vi "GTH-V2.MISC.vi"(7 "CMD":enum16{"All", "ChanA", "ChanB", "Single"}(ring), 8 "Error In":errorcluster caption="错误输入", 9 "ON/FF":bool, 10 "Para":T1(ring), 11 "VISA资源输入":refnum<visa-resource-name>) -> (0 "Error Out":errorcluster caption="错误输出", 2 "CMD Info":string, 3 "OK?":bool)   [LabVIEW 2012, in "Lib_UEL.ATE.lvlib" / "STM32-CoreBD.lvlib"]
uses:
  STM32-CoreBD.lvlib
panel:
  out "Return":string
  # "Version History\nV1.0.0,2015-8-11, 适用于新版GTH-V2硬件."
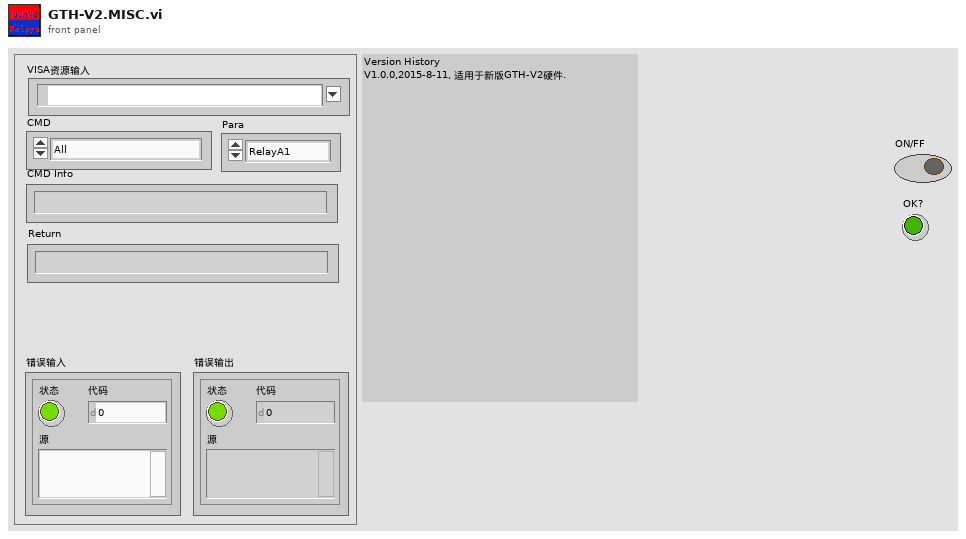
[diagram p1: front panel]
types:
  T1 = enum16{"RelayA1", "RelayA2", "RelayA3", "RelayA4", "RelayA5", "RelayA6", "RelayA7", "RelayA8", "RelayA9", "RelayA10", "RelayB1", "RelayB2", "RelayB3", "RelayB4", "RelayB5", "RelayB6", "RelayB7", "RelayB8", "RelayB9", "RelayB10", "ADC1", "ADC2", "ADC3", "DAC1"}
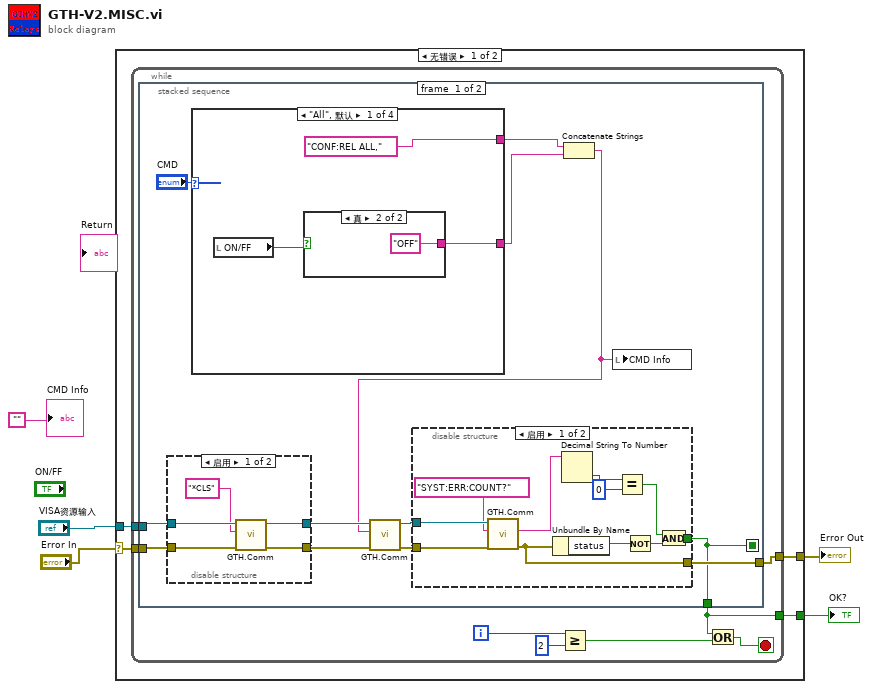
[diagram p0: block diagram]
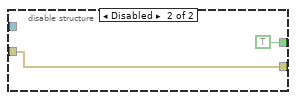
[diagram p2: hidden frame]
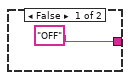
[diagram p4: hidden frame]
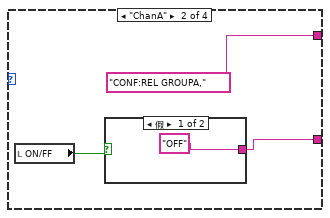
[diagram p5: hidden frame]
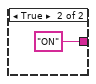
[diagram p6: hidden frame]
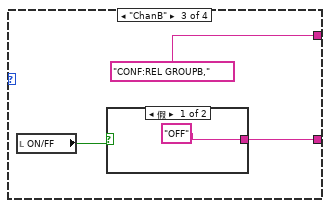
[diagram p7: hidden frame]
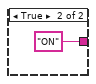
[diagram p8: hidden frame]
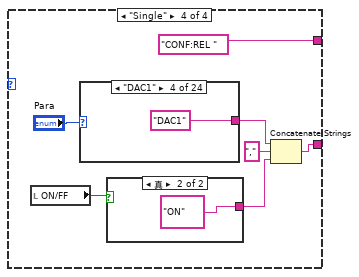
[diagram p9: hidden frame]
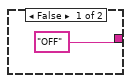
[diagram p10: hidden frame]
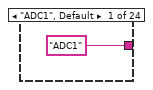
[diagram p11: hidden frame]
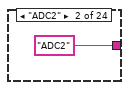
[diagram p12: hidden frame]
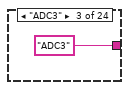
[diagram p13: hidden frame]
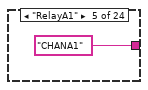
[diagram p14: hidden frame]
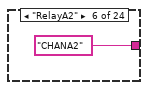
[diagram p15: hidden frame]
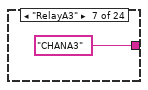
[diagram p16: hidden frame]
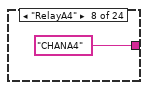
[diagram p17: hidden frame]
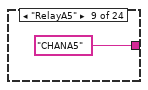
[diagram p18: hidden frame]
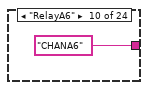
[diagram p19: hidden frame]
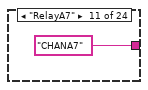
[diagram p20: hidden frame]
diagram:
  n1 = case shown="无错误" "Error In" {
    selector: "Error In" -> [w8 w101]
    tunnel: [w7 w101] -> w5
    tunnel: "VISA资源输入" -> [w9 _]
    tunnel: [w6 FALSE] -> w1
    frame No Error {
      n2 = while {
        tunnel: w9 -> [w17]
        tunnel: w8 -> [w16]
        tunnel: [w15] -> w7
        tunnel: [w10] -> w6
        i -> [w13]
        stop <- w14 stop-if-true
        n3 = stacked-sequence {
          seq-local: [w18 _] -> [_ w98]
          tunnel: w17 -> [w27 _]
          tunnel: w16 -> [w26 _]
          tunnel: [w19 _] -> w15
          tunnel: [w18 _] -> w10
          frame #0 {
            n4 = disable-structure shown="启用" {
              disable-tunnel: w27 -> [w47 w49]
              disable-tunnel: w26 -> [w46 w48]
              disable-tunnel: [w44 w49] -> w25
              disable-tunnel: [w43 w48] -> w24
              frame Enabled {
                n5 = call "GTH.Comm.vi"("Error In"=w46, "SCPI CMD"="*CLS", "USB Port In"=w47) -> ("Error Out"=w43:errorcluster, "USB Port Out"=w44:refnum<visa-resource-name>)  [unwired: 3 in, 4 out]
              }
              frame Disabled {
              }
            }
            n6 = case shown="\"All\", 默认" "CMD" {
              tunnel: ["CONF:REL ALL," ("字符串") "CONF:REL GROUPA," ("字符串") "CONF:REL GROUPB," ("字符串") "CONF:REL " ("字符串")] -> w23
              tunnel: [w51 w55 w60 w68] -> w28
              frame "All", Default {
                n7 = local read "ON/FF"() -> (w50:bool)
                n8 = case shown="真" w50 {
                  tunnel: ["OFF" ("字符串") "OFF" ("字符串")] -> w51
                  frame False {
                  }
                  frame True {
                  }
                }
              }
              frame "ChanA" {
                n9 = local read "ON/FF"() -> (w56:bool)
                n10 = case shown="假" w56 {
                  tunnel: ["OFF" ("字符串") "ON" ("字符串")] -> w55
                  frame False {
                  }
                  frame True {
                  }
                }
              }
              frame "ChanB" {
                n11 = local read "ON/FF"() -> (w61:bool)
                n12 = case shown="假" w61 {
                  tunnel: ["OFF" ("字符串") "ON" ("字符串")] -> w60
                  frame False {
                  }
                  frame True {
                  }
                }
              }
              frame "Single" {
                n13 = local read "ON/FF"() -> (w69:bool)
                n14 = case shown="\"DAC1\"" "Para" {
                  tunnel: ["ADC1" ("字符串") "ADC2" ("字符串") "ADC3" ("字符串") "DAC1" ("字符串") "CHANA1" ("字符串") "CHANA2" ("字符串") "CHANA3" ("字符串") "CHANA4" ("字符串") "CHANA5" ("字符串") "CHANA6" ("字符串") "CHANA7" ("字符串") "CHANA8" ("字符串") "CHANA9" ("字符串") "CHANA10" ("字符串") "CHANB1" ("字符串") "CHANB2" ("字符串") "CHANB3" ("字符串") "CHANB4" ("字符串") "CHANB5" ("字符串") "CHANB6" ("字符串") "CHANB7" ("字符串") "CHANB8" ("字符串") "CHANB9" ("字符串") "CHANB10" ("字符串")] -> w67
                  frame "ADC1", Default {
                  }
                  frame "ADC2" {
                  }
                  frame "ADC3" {
                  }
                  frame "DAC1" {
                  }
                  frame "RelayA1" {
                  }
                  frame "RelayA2" {
                  }
                  frame "RelayA3" {
                  }
                  frame "RelayA4" {
                  }
                  frame "RelayA5" {
                  }
                  frame "RelayA6" {
                  }
                  frame "RelayA7" {
                  }
                  frame "RelayA8" {
                  }
                  frame "RelayA9" {
                  }
                  frame "RelayA10" {
                  }
                  frame "RelayB1" {
                  }
                  frame "RelayB2" {
                  }
                  frame "RelayB3" {
                  }
                  frame "RelayB4" {
                  }
                  frame "RelayB5" {
                  }
                  frame "RelayB6" {
                  }
                  frame "RelayB7" {
                  }
                  frame "RelayB8" {
                  }
                  frame "RelayB9" {
                  }
                  frame "RelayB10" {
                  }
                }
                n15 = case shown="真" w69 {
                  tunnel: ["OFF" ("字符串") "ON" ("字符串")] -> w66
                  frame False {
                  }
                  frame True {
                  }
                }
                n16 = Concatenate Strings(w67, "," ("字符串"), w66) -> (w68:string)
              }
            }
            n17 = Concatenate Strings(w23, w28) -> (w22:string)
            n18 = call "GTH.Comm.vi"("Error In"=w24, "SCPI CMD"=w22, "USB Port In"=w25) -> ("Error Out"=w20:errorcluster, "USB Port Out"=w21:refnum<visa-resource-name>)  [unwired: 3 in, 4 out]
            n19 = disable-structure shown="启用" {
              disable-tunnel: w21 -> [w40 _]
              disable-tunnel: w20 -> [w39 w42]
              disable-tunnel: [w34 w42] -> w19
              disable-tunnel: [w30 TRUE] -> w18
              frame Enabled {
                n20 = call "GTH.Comm.vi"("Error In"=w39, "SCPI CMD"="SYST:ERR:COUNT?", "USB Port In"=w40) -> ("Error Out"=w34:errorcluster, "Return"=w37:string)  [unwired: 3 in, 4 out]
                n21 = Unbundle By Name(w34) -> ("status"=w33:bool)
                n22 = Decimal String To Number(string=w37) -> (number=w36:i32)  [unwired: 2 in, 1 out]
                n23 = Equal?(x=w36, y=0) -> (x = y?=w31:bool)
                n24 = Not(x=w33) -> (.not. x?=w32:bool)
                n25 = And(x=w31, y=w32) -> (x .and. y?=w30:bool)
              }
              frame Disabled {
              }
            }
            n26 = local write "CMD Info"(w22) -> ()
          }
          frame #1 {
            n27 = case shown="假" w98 {
              frame False {
                n28 = Wait (ms)(milliseconds to wait=u32 800 ("等待时间（毫秒）")) -> ()  [unwired: 1 out]
              }
              frame True {
              }
            }
          }
        }
        n29 = Greater Or Equal?(x=w13, y=2) -> (x >= y?=w11:bool)
        n30 = Or(x=w10, y=w11) -> (x .or. y?=w14:bool)
      }
    }
    frame Error {
    }
  }
  "Error Out" <- w5
  "OK?" <- w1
  "CMD Info" <- ""
